vi "reconfigure channel.vi"(6 "user event":T1, 7 "instance identifier":string, 8 "error in":errorcluster, 9 "line":T2, 10 "Data Access:Engine Configuration":refnum<class "engine configuration.lvclass">, 11 "Shared Library Module configuration in":refnum<class "Shared Library Module configuration.lvclass">) -> (0 "error out":errorcluster, 2 "engine configuration out":refnum<class "engine configuration.lvclass">, 3 "Shared Library Module configuration out":refnum<class "Shared Library Module configuration.lvclass">)   [LabVIEW 2013, in "Shared Library Module editor node.lvclass"]
uses:
  Shared Library Module editor node.lvclass
  <vilib>/NI/Module Execution Interface/Engine Configuration/engine configuration.lvclass
  <vilib>/NI/TBM Modules/CLFN/configuration/Shared Library Module configuration.lvclass
  table line.ctl
  <vilib>/NI/Tag Bus Module Framework/channel/TBM channel.lvclass
  <vilib>/CEF_TreeControl/Node/UserEventRef.ctl
  <vilib>/CEF_TreeControl/Controls/EventCluster.ctl
  <vilib>/NI/Tag Bus/tag/tag descriptor.lvclass/tag descriptor.ctl
  <vilib>/NI/Tag Bus/tag/tag descriptor.lvclass
  <vilib>/CEF_TreeControl/NISE_CEF_TreeControl.lvlib
  <vilib>/CEF_TreeControl/Node/NISE_CEF_Node.lvclass
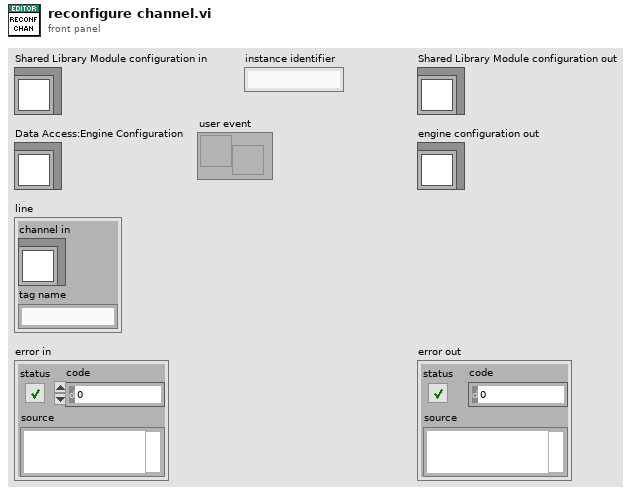
[diagram p1: front panel]
types:
  T1 = typedef "NISE_CEF_Node.lvclass/UserEventRef.ctl" = refnum<user-event>
  T2 = typedef "Shared Library Module editor node.lvclass/table line.ctl" = cluster{"channel in":refnum<class "TBM channel.lvclass">, "tag name":string}
  T3 = typedef "NISE_CEF_TreeControl.lvlib/EventCluster.ctl" = cluster{"command":string, "data":string}
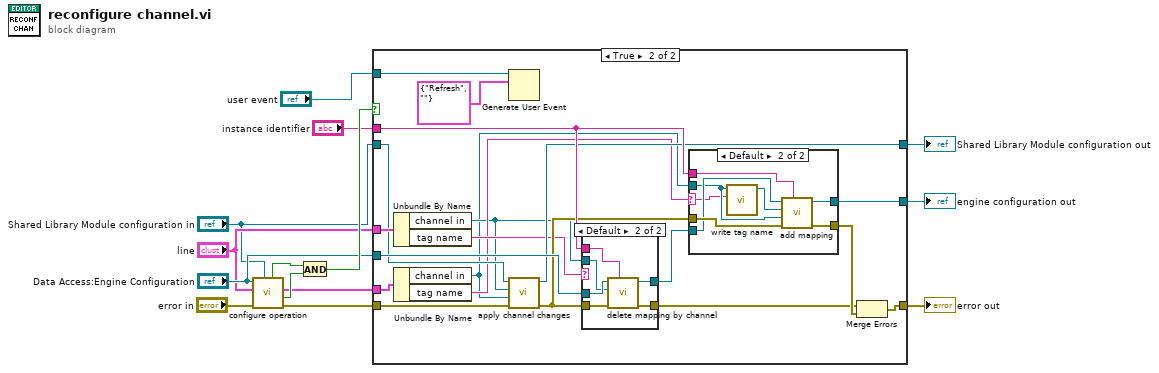
[diagram p0: block diagram]
diagram:
  n1 = call "configure operation.vi"("Shared Library Module configuration in"="Shared Library Module configuration in", "error in"="error in", "line item in"="line", "engine configuration in"="Data Access:Engine Configuration") -> ("error out"=w6:errorcluster, "success"=w10:bool, "line item out"=w3:T2, "changed"=w11:bool)  [unwired: 4 in]
  n2 = And(x=w11, y=w10) -> (x .and. y?=w13:bool)
  n3 = case shown="True" w13 {
    tunnel: [w16 w29] -> w5
    tunnel: [w17 w30] -> w8
    tunnel: "Data Access:Engine Configuration" -> [w17 w34]
    tunnel: w6 -> [w16 w27]
    tunnel: w3 -> [_ w36]
    tunnel: "Shared Library Module configuration in" -> [w15 w24]
    tunnel: [w15 w26] -> w7
    tunnel: "instance identifier" -> [_ w32]
    tunnel: "line" -> [_ w35]
    tunnel: "user event" -> [_ w18]
    frame False {
    }
    frame True {
      n4 = Unbundle By Name(w35) -> ("channel in"=w21:refnum<class "TBM channel.lvclass">, "tag name"=w23:string)
      n5 = Unbundle By Name(w36) -> ("channel in"=w20:refnum<class "TBM channel.lvclass">, "tag name"=w22:string)
      n6 = Generate User Event(user event=w18, event data cluster=T3 {"command"="Refresh", "data"=""} ("event data")) -> ()  [unwired: 2 in, 2 out]
      n7 = call <vilib>:"apply channel changes.vi"("error in"=w27, "new"=w20, "old"=w21, "Shared Library Module configuration in"=w24) -> ("error out"=w25:errorcluster, "Shared Library Module configuration out"=w26:refnum<class "Shared Library Module configuration.lvclass">)  [unwired: 6 in]
      n8 = case shown="Default" w23 {
        tunnel: w25 -> [w37 w44]
        tunnel: w34 -> [w38 w43]
        tunnel: w21 -> [_ w42]
        tunnel: [w37 w41] -> w28
        tunnel: w32 -> [_ w40]
        tunnel: [w38 w39] -> w31
        frame "" {
        }
        frame Default {
          n9 = call <vilib>:"delete mapping by channel.vi"("owner ID"=w40, "error in"=w44, "channel"=w42, "engine configuration in"=w43) -> ("error out"=w41:errorcluster, "engine configuration out"=w39:refnum<class "engine configuration.lvclass">)  [unwired: 6 in]
        }
      }
      n10 = case shown="Default" w22 {
        selector: w22 -> [_ w47]
        tunnel: w25 -> [w45 w54]
        tunnel: [w45 w53] -> w33
        tunnel: w32 -> [_ w52]
        tunnel: w31 -> [w46 w51]
        tunnel: [w46 w50] -> w30
        tunnel: w20 -> [_ w48]
        frame "" {
        }
        frame Default {
          n11 = call <vilib>:"write tag name.vi"("name"=w47, "system tag in"=w48) -> ("system tag out"=w49:refnum<class "TBM channel.lvclass">)  [unwired: 8 in, 1 out]
          n12 = call <vilib>:"add mapping.vi"("owner ID"=w52, "error in"=w54, "channel"=w48, "tag descriptor"=w49, "engine configuration"=w51) -> ("error out"=w53:errorcluster, "engine configuration out"=w50:refnum<class "engine configuration.lvclass">)  [unwired: 5 in]
        }
      }
      n13 = Merge Errors(w28, w33) -> (w29:errorcluster)
    }
  }
  "engine configuration out" <- w8
  "Shared Library Module configuration out" <- w7
  "error out" <- w5
